vi "Get Variables.vi"(8 "error in (no error)":errorcluster, 11 "Message Popup in":refnum<class "UI Functions.lvclass">) -> (0 "error out":errorcluster, 2 "Variables":variant, 3 "Message Popup out":refnum<class "UI Functions.lvclass">)   [LabVIEW 2019, in "UI Functions.lvclass"]
uses:
  UI Functions.lvclass
  UI Functions.lvclass/UI Functions.ctl
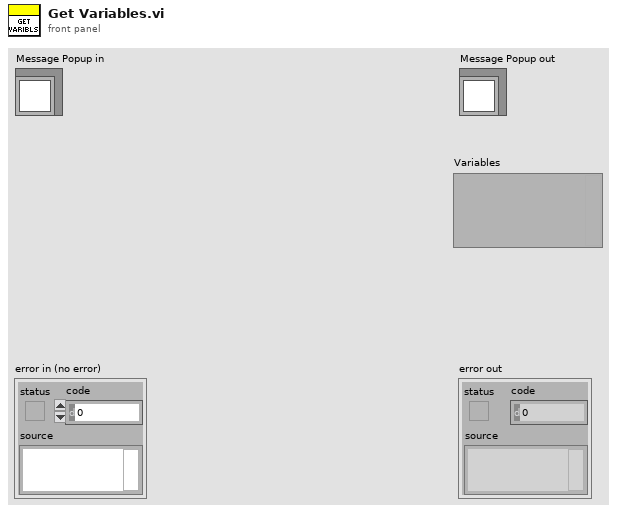
[diagram p1: front panel]
types:
  T1 = typedef "UI Functions.lvclass/Variables.ctl" = cluster{"Message":variant, "T Button":string, "F Button":string}
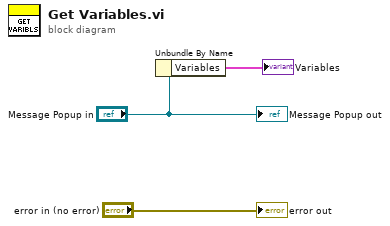
[diagram p0: block diagram]
diagram:
  n1 = Unbundle By Name("Message Popup in") -> ("Variables"=→"Variables":T1)
  "error out" <- "error in (no error)"
  "Message Popup out" <- "Message Popup in"
